vi "ActionVIOnCompile.vi"(8 "error in (no error)":errorcluster, 11 "Device Item Ref in":T1 format="%.0x") -> (0 "error out":errorcluster)   [LabVIEW 2020, in "Communication Bus Template System Explorer.lvlib" / "Implementation.lvlib"]
uses:
  Implementation.lvlib
  <vilib>/NI VeriStand/Custom Device API/Custom Device API.lvlib
  <vilib>/NI VeriStand/Custom Device API/Data Reference.ctl
  <vilib>/NI VeriStand/Custom Device API/Block Data Reference.ctl
  <vilib>/NI VeriStand/Custom Device API/Set Item Property (Variant).vi
  Engine/Interfaces/Execution Unit Factory/Execution Unit Factory.lvclass
  Engine/Implementation/Execution Unit Factory/Execution Unit Factory.lvclass
  Engine/Custom Device/Inline Execution Unit Compiled Information.ctl
  Engine/Custom Device/Custom Device.lvlib
  Engine/Custom Device/Asynchronous Execution Unit Compiled Information.ctl
  Engine/Custom Device/Compiled.Settings.ctl
  C:/Dev/GitHub/niveristand-communications-bus-template/Source/Custom Device Support/Engine/Implementation/Execution Unit Factory/Execution Unit Factory.lvclass
  C:/Dev/GitHub/niveristand-communications-bus-template/Source/Custom Device Support/Engine/Interfaces/Execution Unit Factory/Execution Unit Factory.lvclass
  <vilib>/NI VeriStand/Custom Device API/Custom Device Item Ref.ctl
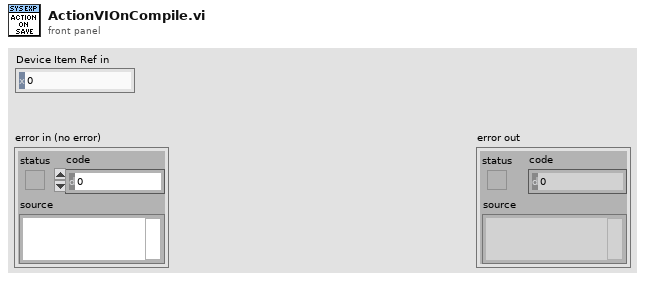
[diagram p1: front panel]
types:
  T1 = typedef "Custom Device API.lvlib/Custom Device Item Ref.ctl" = u64
  T2 = typedef "Communication Bus Template Engine.lvlib/Custom Device.lvlib/Compiled.Settings.ctl" = cluster{"Name":string, "Inline Execution Unit Compiled Information":T3[], "Asynchronous Execution Unit Compiled Information":T6[]}
  T3 = typedef "Communication Bus Template Engine.lvlib/Custom Device.lvlib/Inline Execution Unit Compiled Information.ctl" = cluster{"Flattened Execution Unit":string, "Incoming Buffer":dbl[], "Outgoing Buffer":dbl[], "Incoming Data References":T4[], "Outgoing Data References":T5[]}
  T4 = typedef "Custom Device API.lvlib/Data Reference.ctl" = i32
  T5 = typedef "Custom Device API.lvlib/Block Data Reference.ctl" = cluster{"Data Reference":T4, "Offset":u64, "Length":u64}
  T6 = typedef "Communication Bus Template Engine.lvlib/Custom Device.lvlib/Asynchronous Execution Unit Compiled Information.ctl" = cluster{"Flattened Execution Unit":string, "Incoming Channel Group Name":string, "Outgoing Channel Group Name":string}
  T7 = typedef "Custom Device API.lvlib/Custom Device Item Info.ctl" = cluster{"Name":string, "Is Channel":bool, "GUID":string, "Is Waveform":bool}
  T8 = typedef "Communication Bus Template Engine.lvlib/Interfaces.lvlib/Execution Unit Information.ctl" = cluster{"Execution Unit":refnum<class "Execution Unit.lvclass">, "Incoming Channels":T1[], "Outgoing Channels":T1[]}
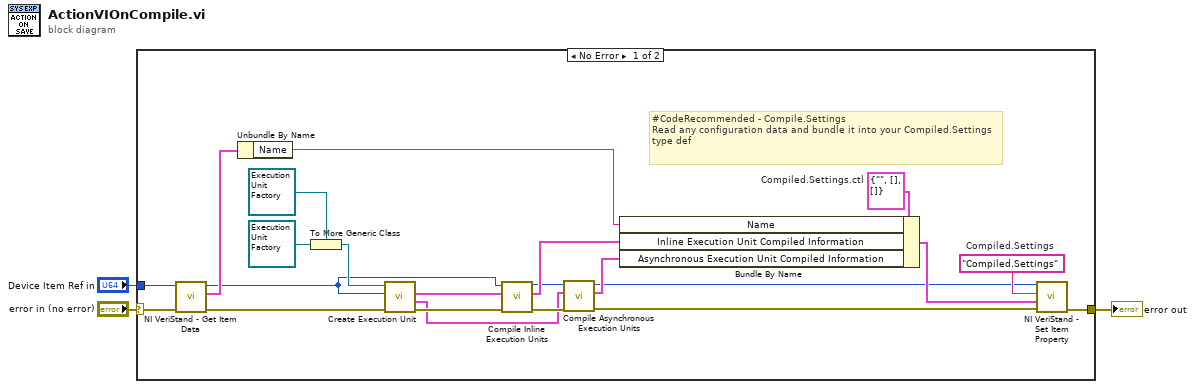
[diagram p0: block diagram]
diagram:
  n1 = case shown="No Error" "error in (no error)" {
    selector: "error in (no error)" -> [w20 w26]
    tunnel: [w23 w26] -> w2
    tunnel: "Device Item Ref in" -> [w17 _]
    frame No Error {
      w21 = T2 {"Name"="", "Inline Execution Unit Compiled Information"=[], "Asynchronous Execution Unit Compiled Information"=[]}  # Compiled.Settings.ctl
      w25 = "Compiled.Settings"  # Compiled.Settings
      # "#CodeRecommended - Compile.Settings\nRead any configuration data and bundle it into your Compiled.Settings type def"
      n2 = call <vilib>:"NI VeriStand - Get Item Data.vi"("error in (no error)"=w20, "Item Ref in"=w17) -> ("error out"=w9:errorcluster, "Item Info"=w22:T7, "Item Ref out"=w8:T1)  [unwired: 6 in, 1 out]
      n3 = Unbundle By Name(w22) -> ("Name"=w18:string)
      n4 = To More Generic Class(target class=refnum<class "Execution Unit Factory.lvclass"> refnum ("Communication Bus Template Interfaces:Interfaces.lvlib:Execution Unit Factory.lvclass"), reference=refnum<class "Execution Unit Factory.lvclass"> refnum ("Communication Bus Template Interfaces:Implementation.lvlib:Execution Unit Factory.lvclass")) -> (generic class reference=w16:refnum<class "Execution Unit Factory.lvclass">)
      n5 = call-dynamic "Create Execution Unit.vi"("error in"=w9, "Item Ref"=w8, "Execution Unit Factory in"=w16) -> ("error out"=w19:errorcluster, "Asynchronous Execution Units"=w6:T8[], "Inline Execution Units"=w14:T8[])  [unwired: 5 in, 1 out]
      n6 = call "Compile Inline Execution Units.vi"("error in"=w19, "Inline Execution Units"=w14, "Device Ref in"=w8) -> ("error out"=w13:errorcluster, "Compiled Inline Execution Units"=w15:T3[], "Device Ref out"=w12:T1)  [unwired: 6 in]
      n7 = call "Compile Asynchronous Execution Units.vi"("Device Ref in"=w12, "Asynchronous Execution Units"=w6, "error in"=w13) -> ("Device Ref out"=w7:T1, "Compiled Asynchronous Execution Units"=w11:T6[], "error out"=w10:errorcluster)  [unwired: 5 in]
      n8 = Bundle By Name(cluster=w21, "Name"=w18, "Inline Execution Unit Compiled Information"=w15, "Asynchronous Execution Unit Compiled Information"=w11) -> (w24:T2)
      n9 = call-poly <vilib>:"NI VeriStand - Set Item Property.vi"("error in (no error)"=w10, "Value"=w24, "Property Name"=w25, "Item Ref in"=w7) -> ("error out"=w23:errorcluster)  [unwired: 5 in, 2 out]
    }
    frame Error {
    }
  }
  "error out" <- w2
